vi "monitor1.vi"() -> ()   [LabVIEW 2012]
uses:
  <vilib>/addons/database/Auxilliary.llb/DB Tools Cursor Type.ctl
  <vilib>/addons/database/Connection.llb/DB Tools Open Connec (Path).vi
  <vilib>/addons/database/Connection.llb/Conn Execute.vi
  <vilib>/addons/database/Recordset.llb/Rec Fetch Recordset Data (R).vi
  <vilib>/addons/database/Recordset.llb/Rec Destroy - Connection.vi
  <vilib>/addons/database/_DB Variant To Data/Database Variant To Data.xnode
  <vilib>/addons/database/NI_Database_API.lvlib
panel:
  out "second subarray 2":dbl[](array[numeric])
  out "second subarray":string[](array[string])
  out "first subarray 6":dbl[](array[numeric])
  out "first subarray 5":dbl[](array[knob]) scale=0.0..10.0
  out "first subarray 4":dbl[](array[knob]) scale=100.0..600.0
  out "first subarray 3":string[](array[string])
  out "first subarray 2":string[](array[string])
  out "first subarray":string[](array[string])
  out "ActualData":dbl[](array[numeric])
  in  "Array 4":dbl[](array[numeric])
  out "index of element":i32
  out "Array 3":string[](array[string])
  out "element":dbl
  out "Array 2":i32[](array[numeric])
  out "Machine":string[](array[string])
  out "UPH":dbl[](array[knob]) scale=100.0..600.0 scale format="%#.8g"
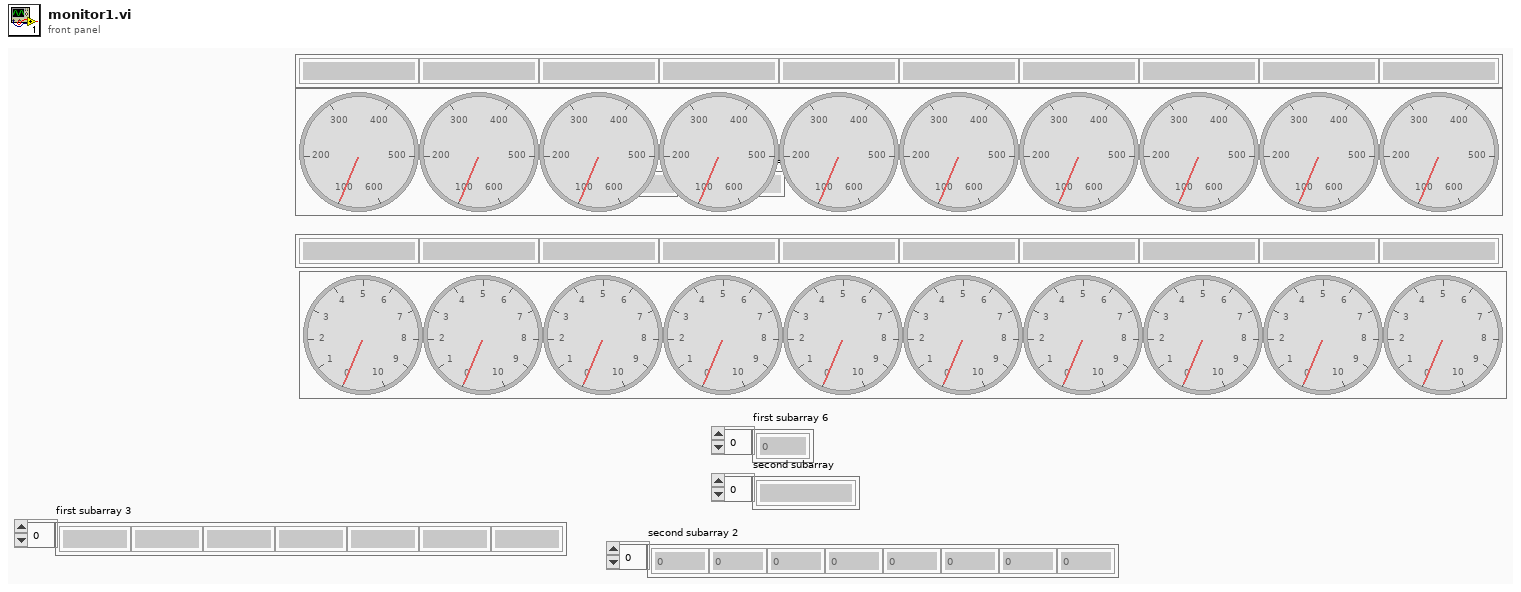
[diagram p1: front panel]
types:
  T1 = typedef "NI_Database_API.lvlib/DB Tools Cursor Type.ctl" = enum16{"forward-only", "keyset", "dynamic", "static"}
  T2 = typedef "NI_Database_API.lvlib/Conn ObjectReference.ctl" = refnum<k1>
  T3 = typedef "NI_Database_API.lvlib/Rec ObjectReference.ctl" = refnum<k1>
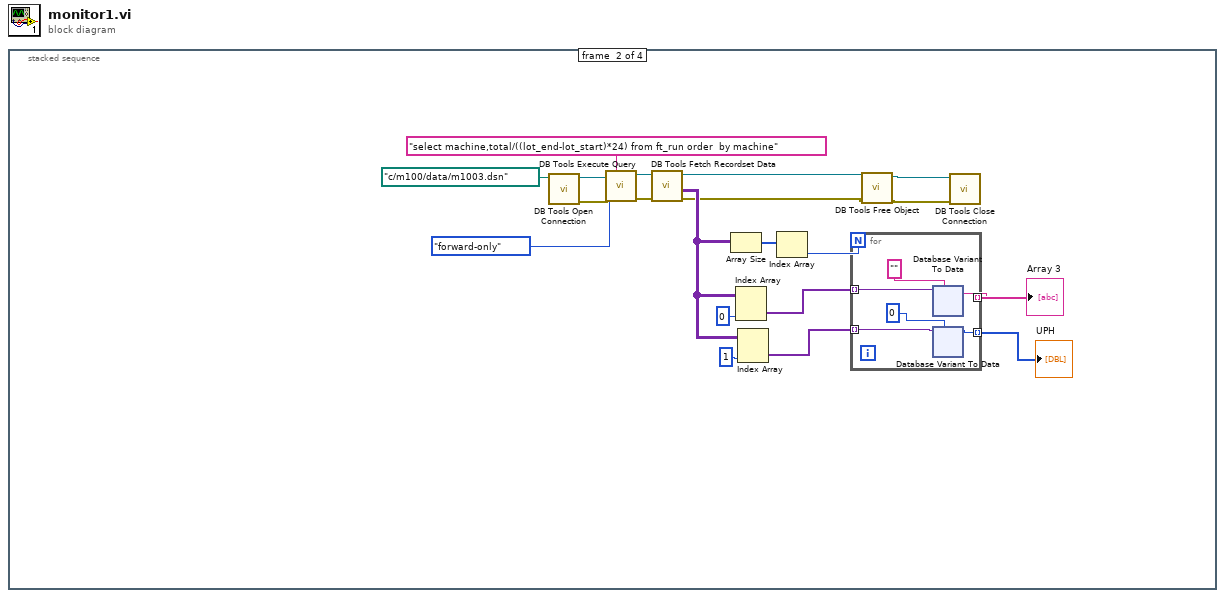
[diagram p0: block diagram]
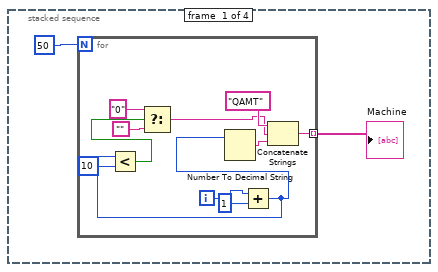
[diagram p2: hidden frame]
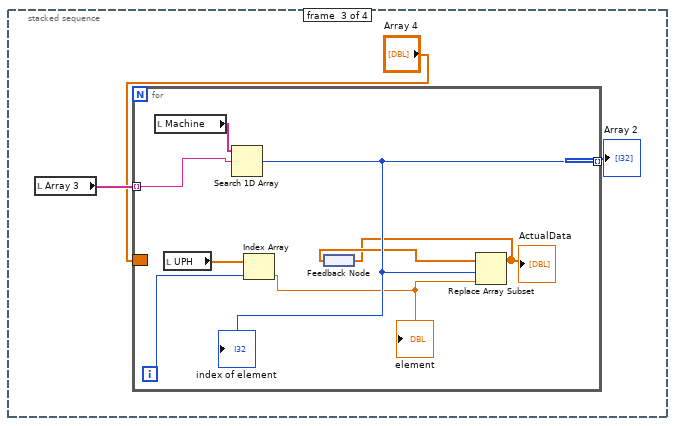
[diagram p3: hidden frame]
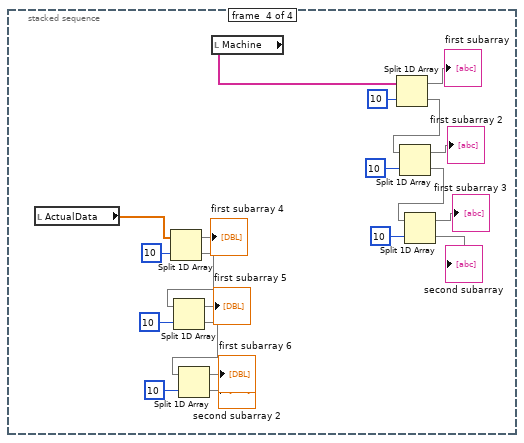
[diagram p4: hidden frame]
diagram:
  n1 = stacked-sequence {
    frame #0 {
      n2 = for {
        N: 50 -> [_]
        tunnel: [w3] -> w2 mode=indexing
        i -> [w12]
        n3 = Add(x=w12, y=1) -> (x+y=w9:i32)
        n4 = Less?(x=w9, y=10) -> (x < y?=w7:bool)
        n5 = Select(t="0", s=w7, f="") -> (s? t:f=w4:string)
        n6 = Number To Decimal String(number=w9) -> (decimal integer string=w10:string)  [unwired: 1 in]
        n7 = Concatenate Strings("QAMT" ("string"), w4, w10) -> (w3:string)
      }
      "Machine" <- w2
    }
    frame #1 {
      n8 = call-poly <vilib>:"DB Tools Open Connection.vi"("connection information"=path "c:/m100/data/m1003.dsn") -> ("error out"=w22:errorcluster, "connection reference"=w23:T2)  [unwired: 7 in]
      n9 = call-poly <vilib>:"DB Tools Execute Query.vi"("error in (no error)"=w22, "cursor type"=DB_Tools_Cursor_Type."forward-only", "SQL query"="select machine,total/((lot_end-lot_start)*24) from ft_run order  by machine", "connection reference"=w23) -> ("error out"=w26:errorcluster, "recordset reference"=w27:T3)  [unwired: 4 in]
      n10 = call-poly <vilib>:"DB Tools Fetch Recordset Data.vi"("error in (no error)"=w26, "recordset reference"=w27) -> ("error out"=w31:errorcluster, "recordset data"=w32:variant[][], "recordset reference out"=w30:T3)  [unwired: 3 in]
      n11 = Array Size(array=w32) -> (size(s)=w16:i32[])
      n12 = Index Array(array=w32, index (col)=0) -> (element=w21:variant[])  [unwired: 1 in]
      n13 = Index Array(array=w32, index (col)=1) -> (element=w19:variant[])  [unwired: 1 in]
      n14 = Index Array(array=w16) -> (element=w17:i32)  [unwired: 1 in]
      n15 = for {
        N: w17 -> [_]
        tunnel: w19 -> [w38] mode=indexing
        tunnel: w21 -> [w39] mode=indexing
        tunnel: [w35] -> w14 mode=indexing
        tunnel: [w34] -> w33 mode=indexing
        n16 = xnode "Database Variant To Data"("database variant"=w39, "type"="") -> ("data"=w34:string)  [unwired: 1 in, 1 out]
        n17 = xnode "Database Variant To Data"("database variant"=w38, "type"=0) -> ("data"=w35:i32)  [unwired: 1 in, 1 out]
      }
      "UPH" <- w14
      "Array 3" <- w33
      n18 = call-poly <vilib>:"DB Tools Free Object.vi"("error in (no error)"=w31, "recordset reference"=w30) -> ("error out"=w29:errorcluster, "connection reference"=w28:T2)  [unwired: 8 in]
      n19 = call <vilib>:"DB Tools Close Connection.vi"("error in (no error)"=w29, "connection reference"=w28) -> ()  [unwired: 5 in, 1 out]
    }
    frame #2 {
      n20 = local read "Array 3"() -> (w105:string[])
      n21 = for {
        tunnel: [w110] -> w106 mode=indexing
        tunnel: w105 -> [w112] mode=indexing
        border: "Array 4" -> [_]
        i -> [w111]
        n22 = local read "Machine"() -> (w114:string[])
        n23 = local read "UPH"() -> (w113:dbl[])
        n24 = Search 1D Array(1D array=w114, element=w112) -> (index of element=w110:i32)  [unwired: 1 in]
        "index of element" <- w110
        n25 = Index Array(array=w113, index=w111) -> (element=w109:dbl)
        "element" <- w109
        n26 = feedback #1() -> (w108:dbl[])
        n27 = Replace Array Subset(array=w108, new element=w109, index=w110) -> (w107:dbl[])
        "ActualData" <- w107
        n28 = feedback-in #1(w107) -> ()
      }
      "Array 2" <- w106
    }
    frame #3 {
      n29 = local read "ActualData"() -> (w120:dbl[])
      n30 = Split 1D Array(array=w120, index=10) -> (first subarray=→"first subarray 4":dbl[], second subarray=w123:dbl[])
      n31 = Split 1D Array(array=w123, index=10) -> (first subarray=→"first subarray 5":dbl[], second subarray=w121:dbl[])
      n32 = Split 1D Array(array=w121, index=10) -> (first subarray=→"first subarray 6":dbl[], second subarray=→"second subarray 2":dbl[])
      n33 = local read "Machine"() -> (w133:string[])
      n34 = Split 1D Array(array=w133, index=10) -> (first subarray=→"first subarray":string[], second subarray=w129:string[])
      n35 = Split 1D Array(array=w129, index=10) -> (first subarray=→"first subarray 2":string[], second subarray=w126:string[])
      n36 = Split 1D Array(array=w126, index=10) -> (first subarray=→"first subarray 3":string[], second subarray=→"second subarray":string[])
    }
  }
